vi "Calibrate (Set).vi"(6 "ISOBUS address":T3=-1 caption="ISOBUS address (-1)", 8 "error in":errorcluster, 11 "Mercury Reference In":T4) -> (0 "error out":errorcluster, 2 "Response":T1, 3 "Mercury Reference Out":T4, 4 "Valid?":T2)   [LabVIEW 2019, in "Mercury iXX.lvlib" / "Heater.lvlib"]
doc: "Calibrates the hardware."
uses:
  Heater.lvlib
  Controls/Mercury Reference.ctl
  CryoTUM_20210311/sub_vi-s/Equipment/Mercury iXX/Public/Controls/Comms Transport Layer.ctl
  Private/Controls/Query Dynamic Reference.ctl
  Controls/ISOBus Address.ctl
  Controls/Is Valid LED.ctl
  Controls/Response String.ctl
  Private/Controls/Command Verbs.ctl
  mercury/Mercury iXX.lvlib
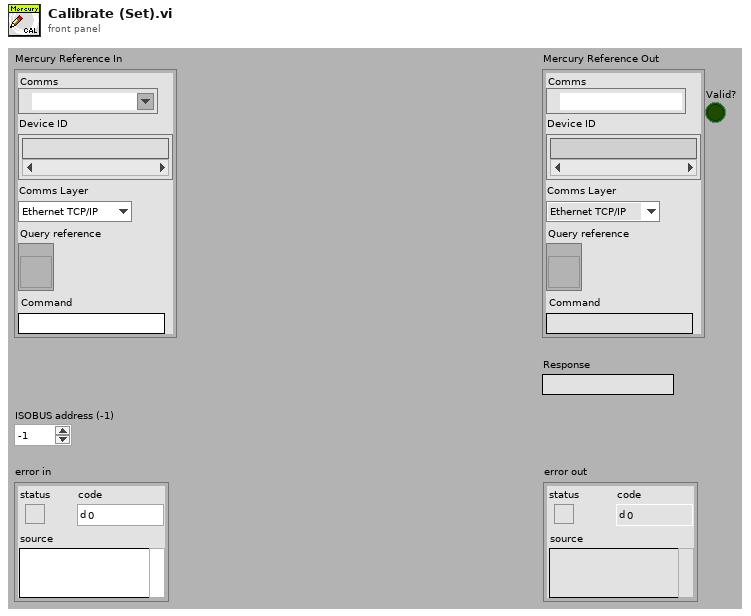
[diagram p1: front panel]
types:
  T1 = typedef "Mercury iXX.lvlib/Response String.ctl" = string
  T2 = typedef "Mercury iXX.lvlib/Is Valid LED.ctl" = bool
  T3 = typedef "Mercury iXX.lvlib/ISOBus Address.ctl" = i32
  T4 = typedef "Mercury iXX.lvlib/Mercury Reference.ctl" = cluster{"Comms":refnum<visa-resource-name>, "Device ID":string[], "Comms Layer":T5, "Command":string, "Query reference":T6}
  T5 = typedef "Mercury iXX.lvlib/Comms Transport Layer.ctl" = enum16{"Ethernet TCP/IP", "USB", "ISOBus - RS-232", "GPIB"}
  T6 = typedef "Mercury iXX.lvlib/Query Dynamic Reference.ctl" = refnum<vi>
  T7 = typedef "Mercury iXX.lvlib/Command Verbs.ctl" = string
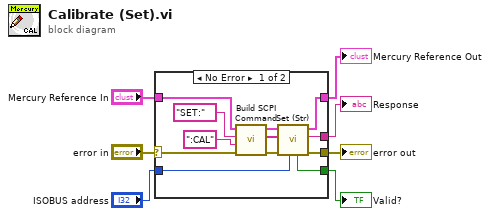
[diagram p0: block diagram]
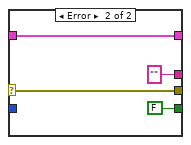
[diagram p2: hidden frame]
diagram:
  n1 = case shown="No Error" "error in" {
    selector: "error in" -> [w8 w23]
    tunnel: [w15 w22] -> w7
    tunnel: [w14 T1 "" ("Response")] -> w6
    tunnel: [w13 T2 FALSE ("Valid?")] -> w5
    tunnel: [w12 w23] -> w4
    tunnel: "ISOBUS address" -> [w11 _]
    tunnel: "Mercury Reference In" -> [w10 w22]
    frame No Error {
      n2 = call "Build SCPI Command.vi"("error in"=w8, "Noun(s)"=":CAL" ("Command"), "Verb"=T7 "SET:", "Mercury Reference In"=w10) -> ("error out"=w16:errorcluster, "SCPI Message(s)"=w17:string[], "Mercury Reference Out"=w18:T4)  [unwired: 5 out]
      n3 = call "Set (Str).vi"("ISOBUS address"=w11, "error in"=w16, "SCPI Message(s)"=w17, "Mercury Reference In"=w18) -> ("error out"=w12:errorcluster, "Response"=w14:T1, "Mercury Reference Out"=w15:T4, "Valid?"=w13:T2)  [unwired: 2 in, 2 out]
    }
    frame Error {
    }
  }
  "Mercury Reference Out" <- w7
  "error out" <- w4
  "Valid?" <- w5
  "Response" <- w6
